vi "Rectify Image Example.vi"() -> ()   [LabVIEW 2020]
uses:
  common/Camera Parameters.ctl
  common/Camera Matrix.ctl
  common/Camera Distortion Coefficients.ctl
  common/Image Size (Integer).ctl
  image/ImageRectifier/ImageRectifier.lvclass/ImageRectifier.ctl
  image/ImageDistorter/ImageDistorter.lvclass/ImageDistorter.ctl
  image/New Image (ARGB).vi
  image/Read Image File (ARGB).vi
  image/Draw Image to Picture (ARGB).vi
  image/ImageRectifier/Rectify Image (ARGB).vi
  image/ImageDistorter/Distort Image (ARGB).vi
  image/New Image (ARGB).vi/3321fa97-f432-4e1e-8db9-a0df79aed21b.vi
  image/ARGB Colour to U32 Pixel Value.vi
  image/Read Image File (ARGB).vi/2358f293-6357-4b7a-bec3-c4e4d03be6e5.vi
  image/Draw Image to Picture (ARGB).vi/8cd07b1b-062e-4fe4-9e87-2eb3dc89fe0e.vi
  image/ImageRectifier/Rectify Image (ARGB).vi/ccc224f2-fea8-4097-85c8-c2b3fe04188f.vi
  image/ImageDistorter/Distort Image (ARGB).vi/ccc224f2-fea8-4097-85c8-c2b3fe04188f.vi
  image/Undistort (ARGB).vi/88690800-d834-48c3-9c45-44dd73aae051.vi
  common/Module Path.vi
  <vilib>/Utility/error.llb/Error Cluster From Error Code.vi
  image/ImageRectifier/ImageRectifier.lvclass
  image/ImageDistorter/ImageDistorter.lvclass
  image/image.lvlib
  common/common.lvlib
panel:
  out "Undistored":picture
  out "New Camera Parameters":T1
  out "Results":T4(array[cluster])
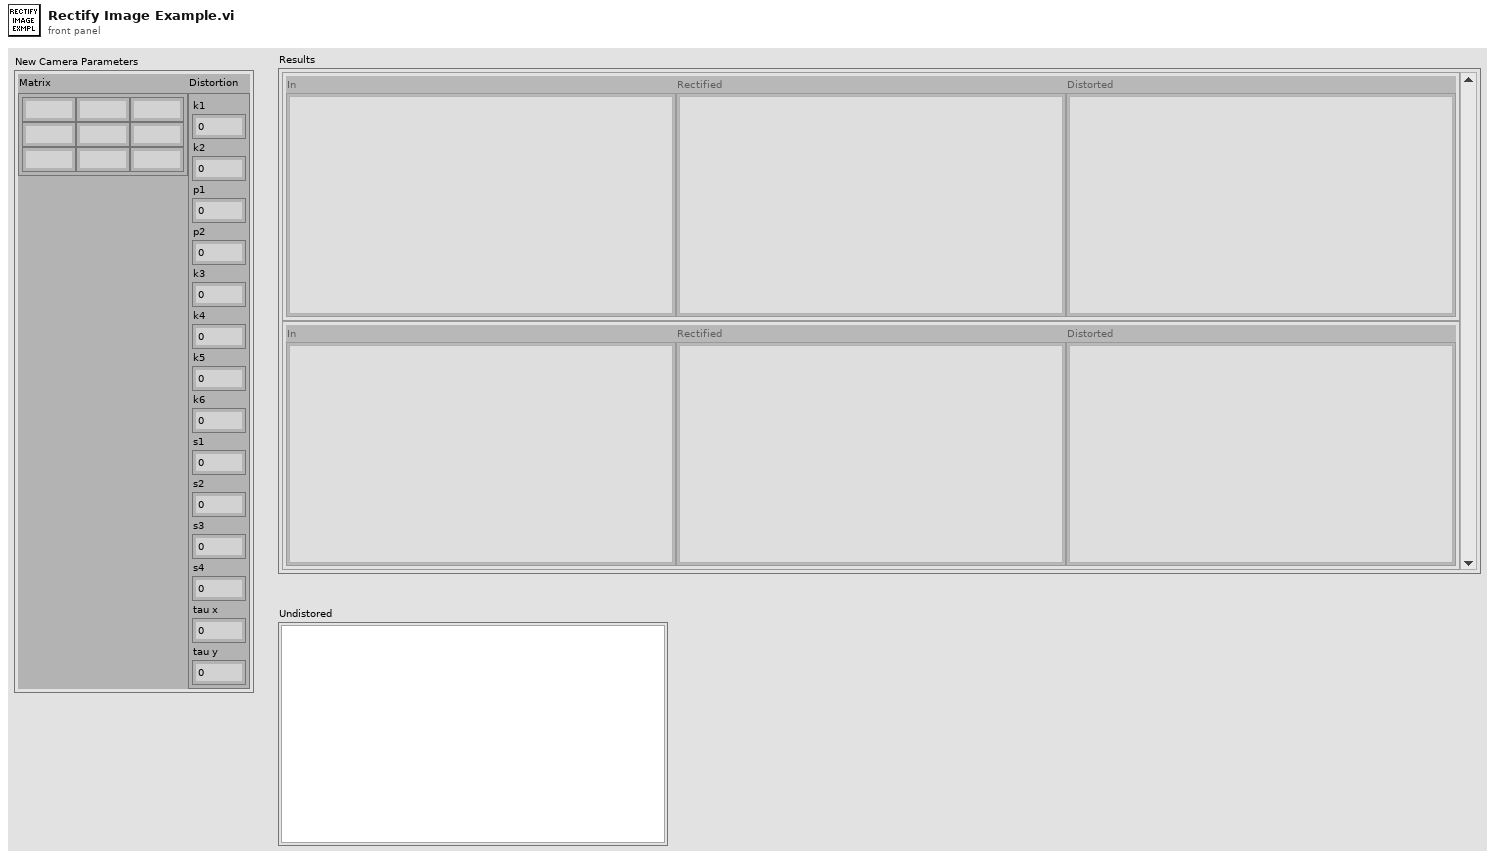
[diagram p1: front panel]
types:
  T1 = typedef "common.lvlib/Camera Parameters.ctl" = cluster{"Matrix":T2, "Distortion":T3}
  T2 = typedef "common.lvlib/Camera Matrix.ctl" = cluster{"m 0,0":dbl, "m 0,1":dbl, "m 0,2":dbl, "m 1,0":dbl, "m 1,1":dbl, "m 1,2":dbl, "m 2,0":dbl, "m 2,1":dbl, "m 2,2":dbl}
  T3 = typedef "common.lvlib/Camera Distortion Coefficients.ctl" = cluster{"k1":dbl, "k2":dbl, "p1":dbl, "p2":dbl, "k3":dbl, "k4":dbl, "k5":dbl, "k6":dbl, "s1":dbl, "s2":dbl, "s3":dbl, "s4":dbl, "tau x":dbl, "tau y":dbl}
  T4 = cluster{"In":picture, "Rectified":picture, "Distorted":picture}[]
  T5 = typedef "common.lvlib/Image Size (Integer).ctl" = cluster{"Width":u16, "Height":u16}
  T6 = typedef "image.lvlib/ARGB Image.ctl" = refnum<data-value>
  T7 = cluster{"Picture":picture, "Picture":picture, "Picture":picture}
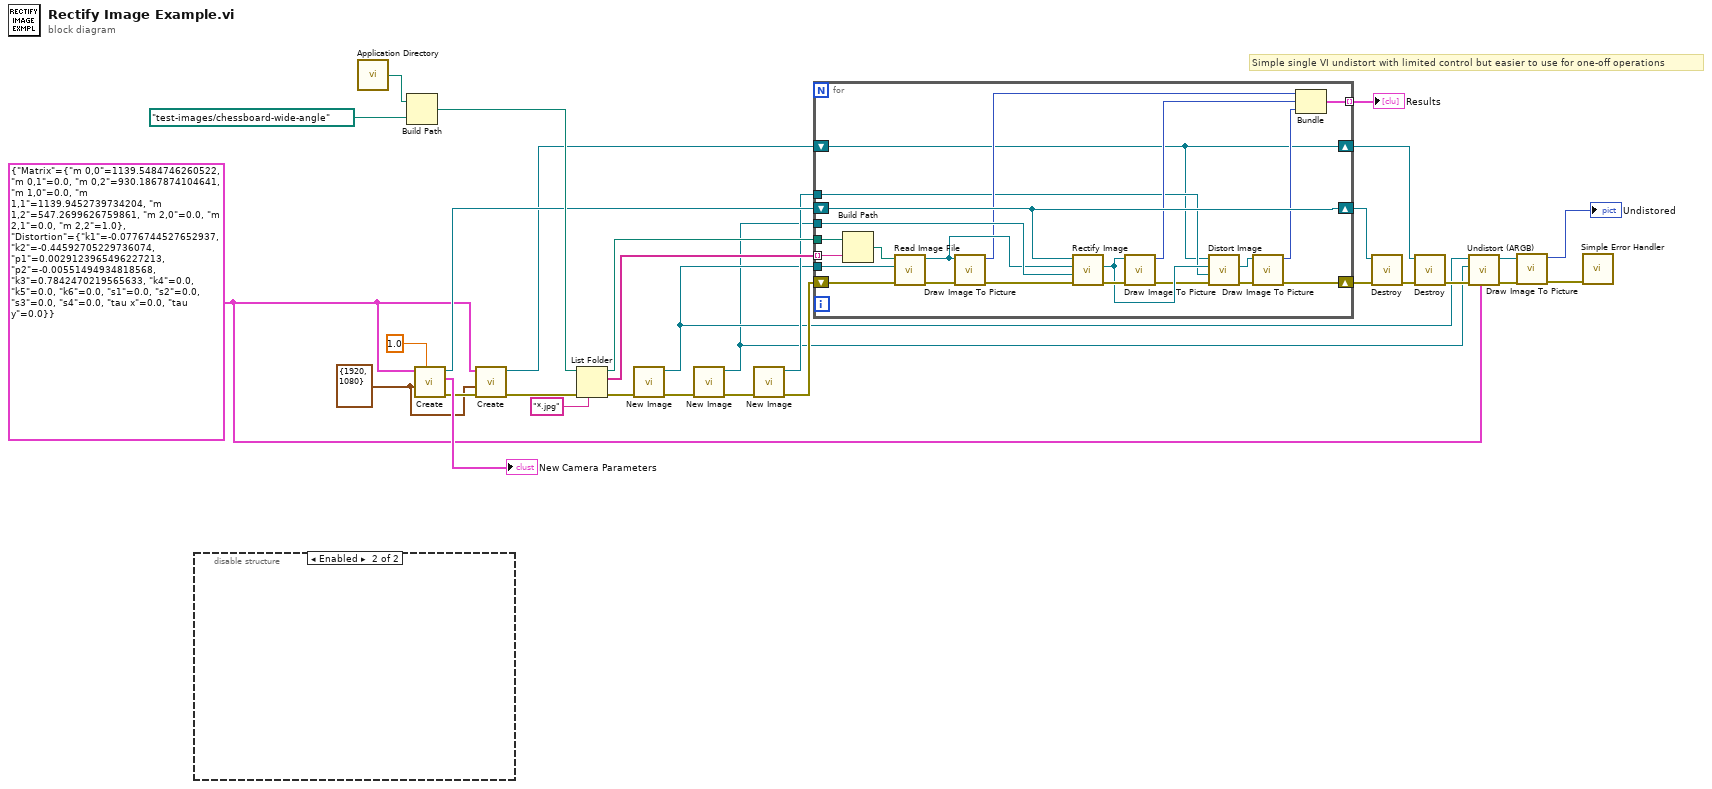
[diagram p0: block diagram]
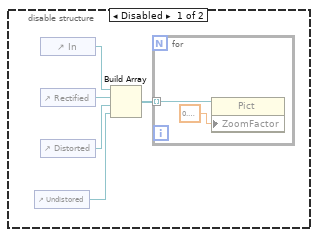
[diagram p2: hidden frame]
diagram:
  w11 = T5 {"Width"=1920, "Height"=1080} ("Image Size")
  w7 = T1 {"Matrix"={"m 0,0"=1139.5484746260522, "m 0,1"=0.0, "m 0,2"=930.1867874104641, "m 1,0"=0.0, "m 1,1"=1139.9452739734204, "m 1,2"=547.2699626759861, "m 2,0"=0.0, "m 2,1"=0.0, "m 2,2"=1.0}, "Distortion"={"k1"=-0.0776744527652937, "k2"=-0.44592705229736074, "p1"=0.0029123965496227213, "p2"=-0.00551494934818568, "k3"=0.7842470219565633, "k4"=0.0, "k5"=0.0, "k6"=0.0, "s1"=0.0, "s2"=0.0, "s3"=0.0, "s4"=0.0, "tau x"=0.0, "tau y"=0.0}} ("Camera Parameters")
  # "Simple single VI undistort with limited control but easier to use for one-off operations"
  n1 = disable-structure shown="Enabled" {
    frame Disabled {
      n2 = control-ref of="Undistored"() -> (w32:refnum<vi>)
      n3 = control-ref of="In"() -> (w36:refnum<vi>)
      n4 = control-ref of="Rectified"() -> (w35:refnum<vi>)
      n5 = control-ref of="Distorted"() -> (w33:refnum<vi>)
      n6 = Build Array(w36, w35, w33, w32) -> (w34:refnum<vi>[])
      n7 = for {
        tunnel: w34 -> [w37] mode=indexing
        n8 = property class="Pict"(reference=w37, "ZoomFactor"=sgl 0.2 ("Zoom Factor")) -> ()  [unwired: 1 in, 2 out]
      }
    }
    frame Enabled {
    }
  }
  n9 = call <vilib>:"Application Directory.vi"() -> ("Application Directory"=w30:path)
  n10 = Build Path(base path=w30, name or relative path=path "test-images/chessboard-wide-angle") -> (appended path=w28:path)
  n11 = call "Create.vi"("Alpha"=1.0, "Image Size"=w11, "Camera Parameters in"=w7) -> ("error out"=w13:errorcluster, "New Camera Parameters"=→"New Camera Parameters":T1, "New ImageRectifier"=w24:refnum<class "ImageRectifier.lvclass">)  [unwired: 4 in, 2 out]
  n12 = call "Create.vi"("error in (no error)"=w13, "Image Size"=w11, "Camera Parameters in"=w7) -> ("error out"=w12:errorcluster, "New ImageDistorter"=w14:refnum<class "ImageDistorter.lvclass">)  [unwired: 7 in]
  n13 = List Folder(path=w28, pattern="*.jpg", error in=w12) -> (path out=w27:path, filenames=w26:string[], error out=w23:errorcluster)  [unwired: 1 in, 1 out]
  n14 = call-poly "New Image.vi"("error in (no error)"=w23) -> ("error out"=w22:errorcluster, "New ARGB Image"=w6:T6)  [unwired: 9 in]
  n15 = call-poly "New Image.vi"("error in (no error)"=w22) -> ("error out"=w17:errorcluster, "New ARGB Image"=w5:T6)  [unwired: 9 in]
  n16 = call-poly "New Image.vi"("error in (no error)"=w17) -> ("error out"=w16:errorcluster, "New ARGB Image"=w15:T6)  [unwired: 9 in]
  n17 = for {
    tunnel: w27 -> [w60]
    tunnel: w26 -> [w59] mode=indexing
    shift-right: [w43] -> w19
    shift-left: w16 -> [w55]
    shift-right: [w57] -> w21
    shift-left: w24 -> [w57]
    tunnel: w6 -> [w56]
    tunnel: w5 -> [w54]
    tunnel: [w47] -> w20 mode=indexing
    tunnel: w15 -> [w45]
    shift-right: [w39] -> w9
    shift-left: w14 -> [w39]
    n18 = Build Path(base path=w60, name or relative path=w59) -> (appended path=w58:path)
    n19 = call-poly "Read Image File.vi"("error in (no error)"=w55, "ARGB Image Destination"=w56, "Filepath"=w58) -> ("error out"=w52:errorcluster, "ARGB Image Destination (duplicate)"=w53:T6)  [unwired: 7 in]
    n20 = call-poly "Draw Image To Picture.vi"("error in (no error)"=w52, "ARGB Image Source"=w53) -> ("error out"=w51:errorcluster, "Picture"=w50:picture)  [unwired: 8 in]
    n21 = call-poly "Rectify Image.vi"("error in (no error)"=w51, "ARGB Image Destination"=w54, "ARGB Image Source"=w53, "ImageRectifier"=w57) -> ("error out"=w49:errorcluster, "ARGB Image Destination (duplicate)"=w46:T6)  [unwired: 5 in, 1 out]
    n22 = call-poly "Draw Image To Picture.vi"("error in (no error)"=w49, "ARGB Image Source"=w46) -> ("error out"=w44:errorcluster, "Picture"=w48:picture)  [unwired: 8 in]
    n23 = call-poly "Distort Image.vi"("error in (no error)"=w44, "ARGB Image Destination"=w45, "ARGB Image Source"=w46, "ImageDistorter"=w39) -> ("error out"=w42:errorcluster, "ARGB Image Destination (duplicate)"=w41:T6)  [unwired: 5 in, 1 out]
    n24 = call-poly "Draw Image To Picture.vi"("error in (no error)"=w42, "ARGB Image Source"=w41) -> ("error out"=w43:errorcluster, "Picture"=w40:picture)  [unwired: 8 in]
    n25 = Bundle("Picture"=w50, "Picture"=w48, "Picture"=w40) -> (w47:T7)  [unwired: 1 in]
  }
  "Results" <- w20
  n26 = call "Destroy.vi"("error in (no error)"=w19, "ImageRectifier in"=w21) -> ("error out"=w10:errorcluster)  [unwired: 9 in]
  n27 = call "Destroy.vi"("error in (no error)"=w10, "ImageRectifier in"=w9) -> ("error out"=w8:errorcluster)  [unwired: 9 in]
  n28 = call "Undistort (ARGB).vi"("Camera Parameters"=w7, "error in (no error)"=w8, "ARGB Image Destination"=w5, "ARGB Image Source"=w6) -> ("error out"=w4:errorcluster, "ARGB Image Destination (duplicate)"=w3:T6)  [unwired: 6 in]
  n29 = call-poly "Draw Image To Picture.vi"("error in (no error)"=w4, "ARGB Image Source"=w3) -> ("error out"=w1:errorcluster, "Picture"=→"Undistored":picture)  [unwired: 8 in]
  n30 = call <vilib>:"Simple Error Handler.vi"("error in (no error)"=w1) -> ()  [unwired: 4 in, 5 out]
